vi "ParseSummary.vi"(11 "Section":string) -> (0 "UPC":string, 1 "Price":dbl, 2 "Pages":i32, 3 "Description":string, 5 "Title":string)   [LabVIEW 2022 SP3]
uses:
  <vilib>/Utility/error.llb/Trim Whitespace One-Sided.vi
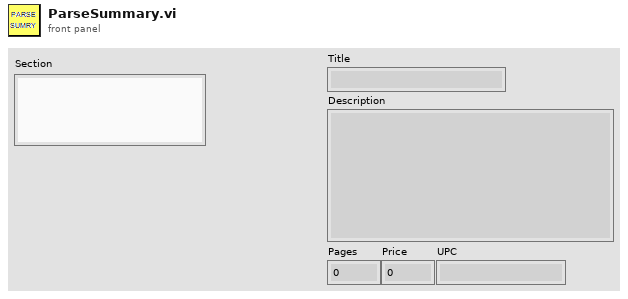
[diagram p1: front panel]
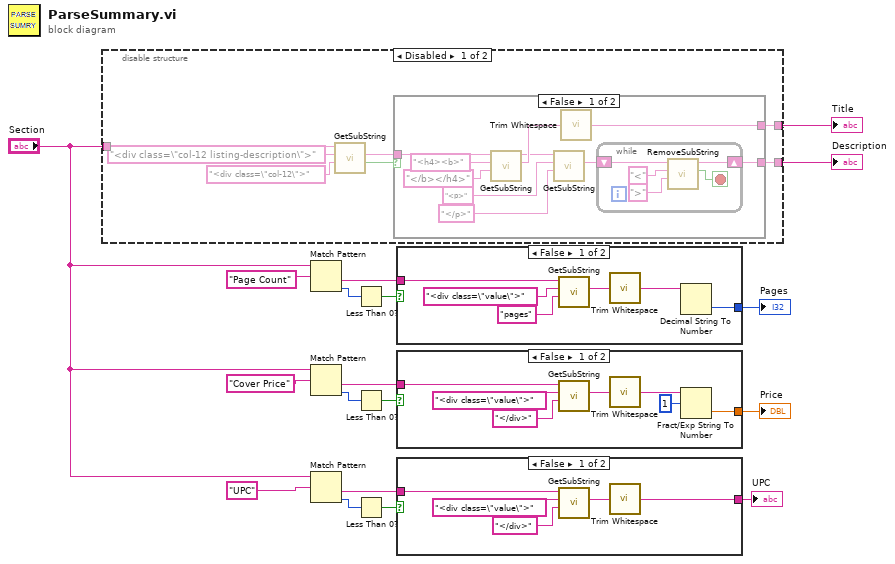
[diagram p0: block diagram]
diagram:
  n1 = disable-structure shown="Disabled" {
    disable-tunnel: [w21 _] -> w18
    disable-tunnel: [w20 _] -> w17
    disable-tunnel: "Section" -> [w19 _]
    frame Disabled {
      n2 = call "GetSubString.vi"("End Search"="<div class=\"col-12\">" ("Start Search"), "Start Search"="<div class=\"col-12 listing-description\">", "String In"=w19) -> ("Not Found?"=w23:bool, "Match"=w22:string)  [unwired: 6 in, 1 out]
      n3 = case shown="False" w23 {
        tunnel: w22 -> [w35 _]
        tunnel: [w31 _] -> w21
        tunnel: [w26 _] -> w20
        frame False {
          n4 = call "GetSubString.vi"("End Search"="</b></h4>", "Start Search"="<h4><b>", "String In"=w35) -> ("Match"=w32:string, "Following String Out"=w30:string)  [unwired: 6 in, 1 out]
          n5 = call "GetSubString.vi"("End Search"="</p>" ("Start Search"), "Start Search"="<p>", "String In"=w30) -> ("Match"=w27:string)  [unwired: 6 in, 2 out]
          n6 = call <vilib>:"Trim Whitespace.vi"("string"=w32) -> ("trimmed string"=w31:string)  [unwired: 1 in]
          n7 = while {
            shift-right: [w36] -> w26
            shift-left: w27 -> [w39]
            stop <- w40 stop-if-true
            n8 = call "RemoveSubString.vi"("Sub End"=">", "Sub Start"="<", "String In"=w39) -> ("Not Found?"=w40:bool, "String Out"=w36:string)  [unwired: 7 in]
          }
        }
        frame True {
        }
      }
    }
    frame Enabled {
    }
  }
  "Title" <- w18
  "Description" <- w17
  n9 = Match Pattern(string="Section", regular expression="Page Count") -> (after substring=w13:string, offset past match=w15:i32)  [unwired: 1 in, 2 out]
  n10 = Match Pattern(string="Section", regular expression="Cover Price") -> (after substring=w10:string, offset past match=w8:i32)  [unwired: 1 in, 2 out]
  n11 = Match Pattern(string="Section", regular expression="UPC") -> (after substring=w3:string, offset past match=w5:i32)  [unwired: 1 in, 2 out]
  n12 = Less Than 0?(x=w15) -> (x < 0?=w14:bool)
  n13 = Less Than 0?(x=w8) -> (x < 0?=w9:bool)
  n14 = Less Than 0?(x=w5) -> (x < 0?=w4:bool)
  n15 = case shown="False" w14 {
    tunnel: w13 -> [w46 _]
    tunnel: [w42 _] -> w12
    frame False {
      n16 = call "GetSubString.vi"("End Search"="pages", "Start Search"="<div class=\"value\">", "String In"=w46) -> ("Match"=w43:string)  [unwired: 6 in, 2 out]
      n17 = call <vilib>:"Trim Whitespace.vi"("string"=w43) -> ("trimmed string"=w41:string)  [unwired: 1 in]
      n18 = Decimal String To Number(string=w41) -> (number=w42:i32)  [unwired: 2 in, 1 out]
    }
    frame True {
    }
  }
  "Pages" <- w12
  n19 = case shown="False" w9 {
    tunnel: w10 -> [w53 _]
    tunnel: [w49 _] -> w11
    frame False {
      n20 = call "GetSubString.vi"("End Search"="</div>", "Start Search"="<div class=\"value\">", "String In"=w53) -> ("Match"=w50:string)  [unwired: 6 in, 2 out]
      n21 = call <vilib>:"Trim Whitespace.vi"("string"=w50) -> ("trimmed string"=w48:string)  [unwired: 1 in]
      n22 = Fract/Exp String To Number(string=w48, offset=1) -> (number=w49:dbl)  [unwired: 2 in, 1 out]
    }
    frame True {
    }
  }
  "Price" <- w11
  n23 = case shown="False" w4 {
    tunnel: w3 -> [w58 _]
    tunnel: [w54 _] -> w1
    frame False {
      n24 = call "GetSubString.vi"("End Search"="</div>", "Start Search"="<div class=\"value\">", "String In"=w58) -> ("Match"=w55:string)  [unwired: 6 in, 2 out]
      n25 = call <vilib>:"Trim Whitespace.vi"("string"=w55) -> ("trimmed string"=w54:string)  [unwired: 1 in]
    }
    frame True {
    }
  }
  "UPC" <- w1
